vi "pralka.vi"() -> ()   [LabVIEW 2023]
uses:
  cluster.ctl
  states.ctl
panel:
  in  "Lid Open":bool
  in  "Drying Enable":bool
  in  "Start":bool
  in  "Dial":i32(knob)=2 scale=0.0..4.0
  out "Power On":bool
  out "Lid open":bool
  in  "stop":bool
  out "Drying":bool
  out "Centrifugation":bool
  out "Pump water out":bool
  out "Motor controll":bool
  out "Water heating":bool
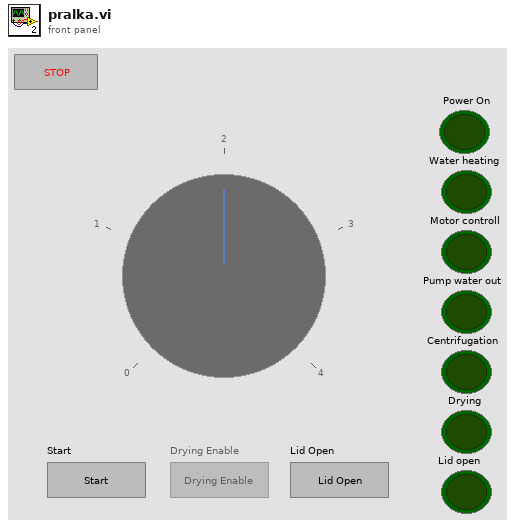
[diagram p1: front panel]
types:
  T1 = typedef "states.ctl" = enum16{"init", "idle", "washing_init", "washing", "wait", "turn_off", "lead_open", "exit"}
  T2 = typedef "cluster.ctl" = cluster{"CurrentTime":timestamp, "CoffeType":enum16{"Cotton", "Silk", "Fast", "Drying"}, "Cluster":cluster{"WaterHeating":i32, "MotorControll":i32, "PumpWaterOut":i32, "Cetrifugation":i32, "Drying":i32}, "TimeToWait":i32, "WashingState":i32, "LidOnTime":dbl}
  T3 = enum8{"Enabled", "Disabled", "Disabled and Grayed Out"}
  T4 = cluster{"WaterHeating":i32, "MotorControll":i32, "PumpWaterOut":i32, "Cetrifugation":i32, "Drying":i32}
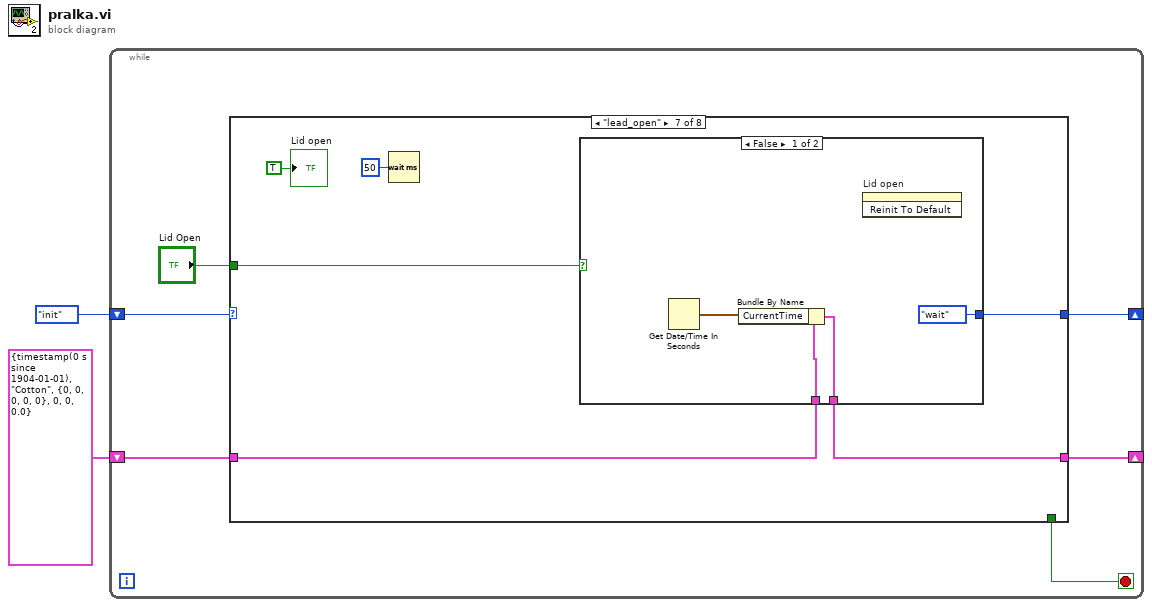
[diagram p0: block diagram]
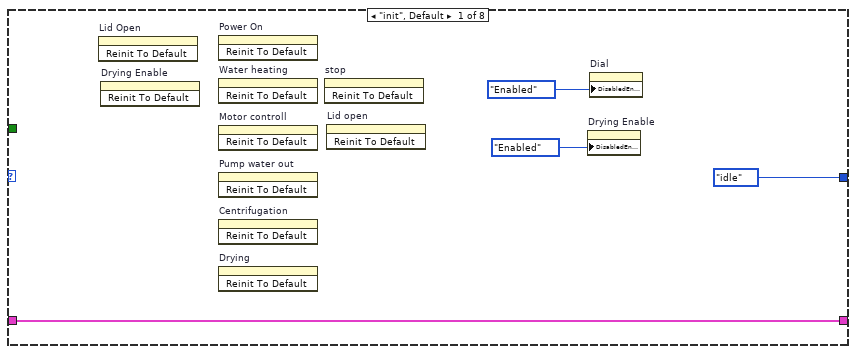
[diagram p2: hidden frame]
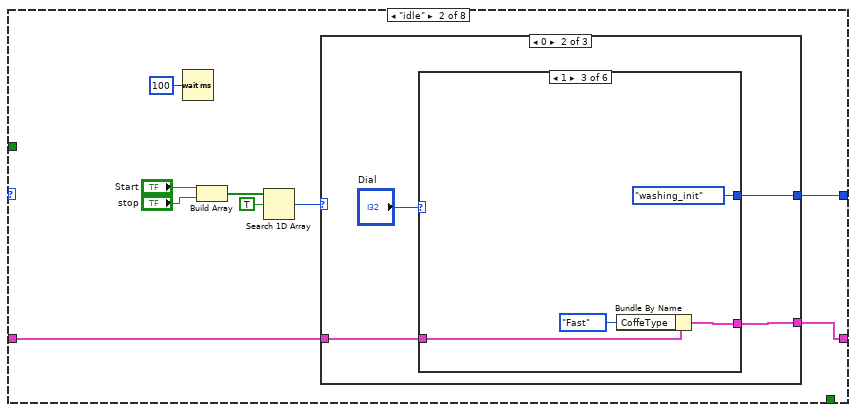
[diagram p3: hidden frame]
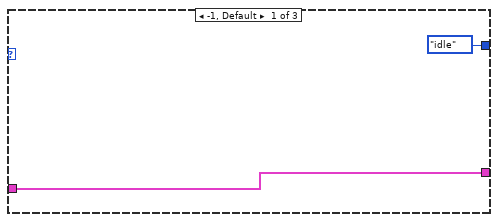
[diagram p4: hidden frame]
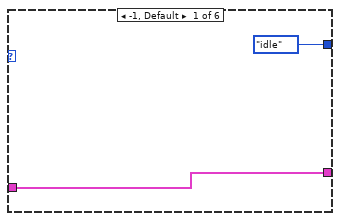
[diagram p5: hidden frame]
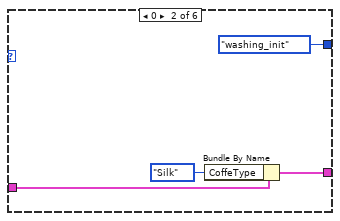
[diagram p6: hidden frame]
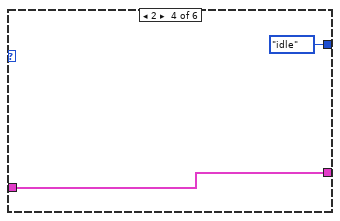
[diagram p7: hidden frame]
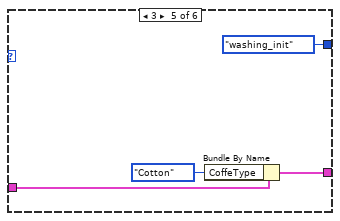
[diagram p8: hidden frame]
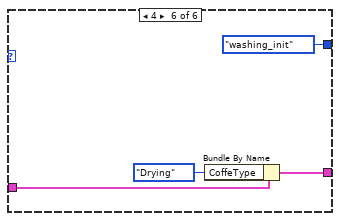
[diagram p9: hidden frame]
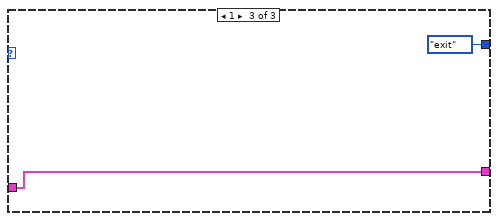
[diagram p10: hidden frame]
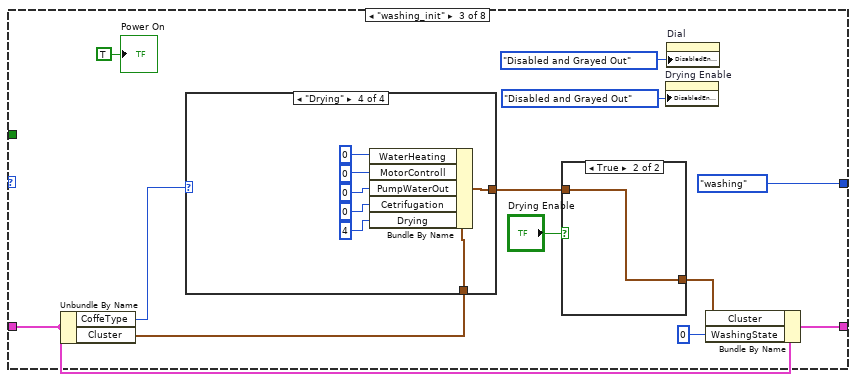
[diagram p11: hidden frame]
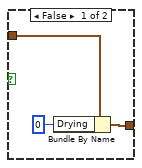
[diagram p12: hidden frame]
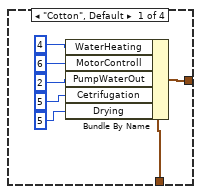
[diagram p13: hidden frame]
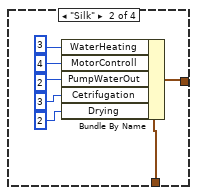
[diagram p14: hidden frame]
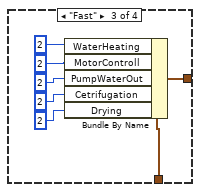
[diagram p15: hidden frame]
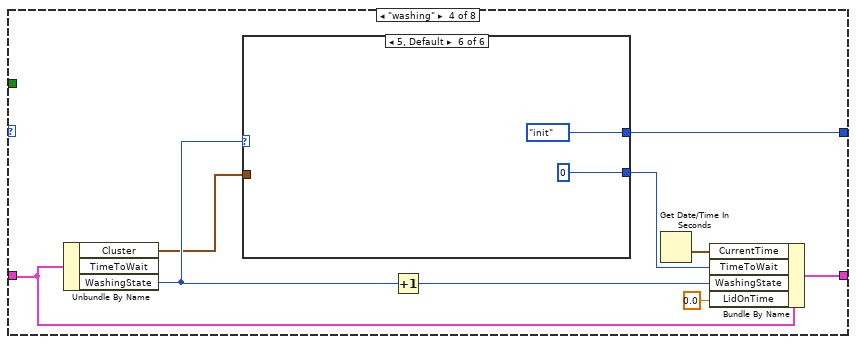
[diagram p16: hidden frame]
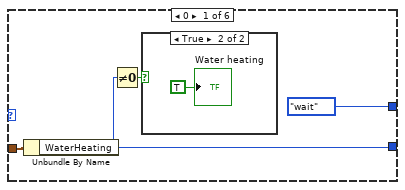
[diagram p17: hidden frame]
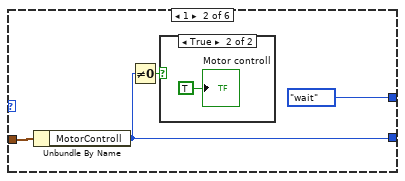
[diagram p19: hidden frame]
diagram:
  n1 = while {
    shift-right: [w7] -> _
    shift-left: states."init" ("Enum") -> [w8]
    shift-right: [w5] -> _
    shift-left: T2 {"CurrentTime"=timestamp(0 s since 1904-01-01), "CoffeType"=enum."Cotton", "Cluster"={"WaterHeating"=0, "MotorControll"=0, "PumpWaterOut"=0, "Cetrifugation"=0, "Drying"=0}, "TimeToWait"=0, "WashingState"=0, "LidOnTime"=0.0} -> [w6]
    stop <- w3 stop-if-true
    n2 = case shown="\"lead_open\"" w8 {
      tunnel: [states."idle" ("Enum") w21 states."washing" ("Enum") w96 w144 states."washing" ("Enum") w174 states."exit" ("Enum")] -> w7
      tunnel: w6 -> [w11 w20 w58 w101 w135 w167 w170 w183]
      tunnel: [w11 w19 w60 w102 w131 w167 w169 w183] -> w5
      tunnel: "Lid Open" -> [_ _ _ _ w136 _ w172 _]
      tunnel: [_ _ _ _ _ _ _ TRUE ("stop")] -> w3
      frame "init", Default {
        n3 = invoke on="Lid Open" class="Bool (strict)" method="Reinit To Default"() -> ()  [unwired: 3 in, 3 out]
        n4 = invoke on="Drying Enable" class="Bool (strict)" method="Reinit To Default"() -> ()  [unwired: 3 in, 3 out]
        n5 = invoke on="Power On" class="Bool (strict)" method="Reinit To Default"() -> ()  [unwired: 3 in, 3 out]
        n6 = invoke on="Water heating" class="Bool (strict)" method="Reinit To Default"() -> ()  [unwired: 3 in, 3 out]
        n7 = invoke on="Motor controll" class="Bool (strict)" method="Reinit To Default"() -> ()  [unwired: 3 in, 3 out]
        n8 = invoke on="Pump water out" class="Bool (strict)" method="Reinit To Default"() -> ()  [unwired: 3 in, 3 out]
        n9 = invoke on="Centrifugation" class="Bool (strict)" method="Reinit To Default"() -> ()  [unwired: 3 in, 3 out]
        n10 = invoke on="Drying" class="Bool (strict)" method="Reinit To Default"() -> ()  [unwired: 3 in, 3 out]
        n11 = invoke on="stop" class="Bool (strict)" method="Reinit To Default"() -> ()  [unwired: 3 in, 3 out]
        n12 = invoke on="Lid open" class="Bool (strict)" method="Reinit To Default"() -> ()  [unwired: 3 in, 3 out]
        n13 = property on="Drying Enable" class="Bool (strict)"("DisabledEnum"=T3."Enabled" ("Disabled")) -> ()  [unwired: 2 in, 2 out]
        n14 = property on="Dial" class="Knob (strict)"("DisabledEnum"=T3."Enabled" ("Disabled")) -> ()  [unwired: 2 in, 2 out]
      }
      frame "idle" {
        n15 = Wait (ms)(milliseconds to wait=u32 100) -> ()  [unwired: 1 out]
        n16 = Build Array("Start", "stop") -> (w15:bool[])
        n17 = Search 1D Array(1D array=w15, element=TRUE) -> (index of element=w13:i32)  [unwired: 1 in]
        n18 = case shown="0" w13 {
          tunnel: [states."idle" ("Enum") w27 states."exit" ("Enum")] -> w21
          tunnel: w20 -> [w22 w26 w49]
          tunnel: [w22 w25 w49] -> w19
          frame -1, Default {
          }
          frame 0 {
            n19 = case shown="1" "Dial" {
              tunnel: [states."idle" ("Enum") states."washing_init" ("Enum") states."washing_init" ("Enum") states."idle" ("Enum") states."washing_init" ("Enum") states."washing_init" ("Enum")] -> w27
              tunnel: w26 -> [w28 w31 w36 w39 w42 w46]
              tunnel: [w28 w32 w37 w39 w43 w47] -> w25
              frame -1, Default {
              }
              frame 0 {
                n20 = Bundle By Name(cluster=w31, "CoffeType"=enum16{"Cotton", "Silk", "Fast", "Drying"}."Silk") -> (w32:T2)
              }
              frame 1 {
                n21 = Bundle By Name(cluster=w36, "CoffeType"=enum16{"Cotton", "Silk", "Fast", "Drying"}."Fast") -> (w37:T2)
              }
              frame 2 {
              }
              frame 3 {
                n22 = Bundle By Name(cluster=w42, "CoffeType"=enum16{"Cotton", "Silk", "Fast", "Drying"}."Cotton") -> (w43:T2)
              }
              frame 4 {
                n23 = Bundle By Name(cluster=w46, "CoffeType"=enum16{"Cotton", "Silk", "Fast", "Drying"}."Drying") -> (w47:T2)
              }
            }
          }
          frame 1 {
          }
        }
      }
      frame "washing_init" {
        n24 = Unbundle By Name(w58) -> ("CoffeType"=w59:enum16{"Cotton", "Silk", "Fast", "Drying"}, "Cluster"=w57:T4)
        n25 = case shown="\"Drying\"" w59 {
          tunnel: [w72 w78 w86 w93] -> w52
          tunnel: w57 -> [w71 w79 w85 w92]
          frame "Cotton", Default {
            n26 = Bundle By Name(cluster=w71, "WaterHeating"=4 ("Espresso"), "MotorControll"=6 ("SteamedMilk"), "PumpWaterOut"=2 ("MilkFoam"), "Cetrifugation"=5 ("ChocolateSyrup"), "Drying"=5 ("WhippedCream")) -> (w72:T4)
          }
          frame "Silk" {
            n27 = Bundle By Name(cluster=w79, "WaterHeating"=3 ("Espresso"), "MotorControll"=4 ("SteamedMilk"), "PumpWaterOut"=2 ("MilkFoam"), "Cetrifugation"=3 ("ChocolateSyrup"), "Drying"=2 ("WhippedCream")) -> (w78:T4)
          }
          frame "Fast" {
            n28 = Bundle By Name(cluster=w85, "WaterHeating"=2 ("Espresso"), "MotorControll"=2 ("SteamedMilk"), "PumpWaterOut"=2 ("MilkFoam"), "Cetrifugation"=2 ("ChocolateSyrup"), "Drying"=2 ("WhippedCream")) -> (w86:T4)
          }
          frame "Drying" {
            n29 = Bundle By Name(cluster=w92, "WaterHeating"=0 ("Espresso"), "MotorControll"=0 ("SteamedMilk"), "PumpWaterOut"=0 ("MilkFoam"), "Cetrifugation"=0 ("ChocolateSyrup"), "Drying"=4 ("WhippedCream")) -> (w93:T4)
          }
        }
        n30 = case shown="True" "Drying Enable" {
          tunnel: [w64 w65] -> w53
          tunnel: w52 -> [w63 w65]
          frame False {
            n31 = Bundle By Name(cluster=w63, "Drying"=0) -> (w64:T4)
          }
          frame True {
          }
        }
        n32 = property on="Drying Enable" class="Bool (strict)"("DisabledEnum"=T3."Disabled and Grayed Out" ("Disabled")) -> ()  [unwired: 2 in, 2 out]
        n33 = property on="Dial" class="Knob (strict)"("DisabledEnum"=T3."Disabled and Grayed Out" ("Disabled")) -> ()  [unwired: 2 in, 2 out]
        n34 = Bundle By Name(cluster=w58, "Cluster"=w53, "WashingState"=0 ("ElementPreparing")) -> (w60:T2)
        "Power On" <- TRUE ("Power On")
      }
      frame "washing" {
        n35 = Unbundle By Name(w101) -> ("Cluster"=w98:T4, "WashingState"=w100:i32)  [unwired: 1 out]
        n36 = case shown="5, Default" w100 {
          tunnel: w98 -> [w106 w111 w116 w121 w126 _]
          tunnel: [w103 w108 w113 w118 w123 0 ("WhippedCream")] -> w97
          tunnel: [states."wait" ("Enum") states."wait" ("Enum") states."wait" ("Enum") states."wait" ("Enum") states."wait" ("Enum") states."init" ("Enum")] -> w96
          frame 0 {
            n37 = Unbundle By Name(w106) -> ("WaterHeating"=w103:i32)
            n38 = Not Equal To 0?(x=w103) -> (x != 0?=w104:bool)
            n39 = case shown="True" w104 {
              frame False {
              }
              frame True {
                "Water heating" <- TRUE ("Espresso")
              }
            }
          }
          frame 1 {
            n40 = Unbundle By Name(w111) -> ("MotorControll"=w108:i32)
            n41 = Not Equal To 0?(x=w108) -> (x != 0?=w109:bool)
            n42 = case shown="True" w109 {
              frame False {
              }
              frame True {
                "Motor controll" <- TRUE ("Steamed Milk")
              }
            }
          }
          frame 2 {
            n43 = Unbundle By Name(w116) -> ("PumpWaterOut"=w113:i32)
            n44 = Not Equal To 0?(x=w113) -> (x != 0?=w114:bool)
            n45 = case shown="True" w114 {
              frame False {
              }
              frame True {
                "Pump water out" <- TRUE ("Milk Foam")
              }
            }
          }
          frame 3 {
            n46 = Unbundle By Name(w121) -> ("Cetrifugation"=w118:i32)
            n47 = Not Equal To 0?(x=w118) -> (x != 0?=w119:bool)
            n48 = case shown="True" w119 {
              frame False {
              }
              frame True {
                "Centrifugation" <- TRUE ("Chocolate Syrup")
              }
            }
          }
          frame 4 {
            n49 = Unbundle By Name(w126) -> ("Drying"=w123:i32)
            n50 = Not Equal To 0?(x=w123) -> (x != 0?=w124:bool)
            n51 = case shown="True" w124 {
              frame False {
              }
              frame True {
                "Drying" <- TRUE ("Whipped Cream")
              }
            }
          }
          frame 5, Default {
          }
        }
        n52 = Increment(x=w100) -> (x+1=w99:i32)
        n53 = Get Date/Time In Seconds() -> (seconds since 1Jan1904=w95:timestamp)
        n54 = Bundle By Name(cluster=w101, "CurrentTime"=w95, "TimeToWait"=w97, "WashingState"=w99, "LidOnTime"=0.0) -> (w102:T2)
      }
      frame "wait" {
        n55 = Unbundle By Name(w135) -> ("CurrentTime"=w142:timestamp, "TimeToWait"=w137:i32, "LidOnTime"=w133:dbl)
        n56 = Get Date/Time In Seconds() -> (seconds since 1Jan1904=w143:timestamp)
        n57 = To Double Precision Float(number=w142) -> (double precision float=w140:dbl)
        n58 = To Double Precision Float(number=w137) -> (double precision float=w139:dbl)
        n59 = To Double Precision Float(number=w143) -> (double precision float=w141:dbl)
        n60 = Subtract(x=w141, y=w140) -> (x-y=w134:dbl)
        n61 = Add(x=w134, y=w133) -> (x+y=w132:dbl)
        n62 = Greater Or Equal?(x=w132, y=w139) -> (x >= y?=w138:bool)
        n63 = local read "stop"() -> (w130:bool)
        n64 = case shown="False" w130 {
          tunnel: [w151 states."exit" ("Enum")] -> w144
          tunnel: w138 -> [w150 _]
          tunnel: w136 -> [w149 _]
          tunnel: w135 -> [w148 w166]
          tunnel: w132 -> [w147 _]
          tunnel: [w146 w166] -> w131
          frame False {
            n65 = case shown="True" w150 {
              tunnel: [w156 states."turn_off" ("Enum")] -> w151
              tunnel: w149 -> [w155 _]
              tunnel: w148 -> [w154 w163]
              tunnel: w147 -> [w153 _]
              tunnel: [w152 w163] -> w146
              frame False {
                n66 = case shown="True" w155 {
                  tunnel: [states."wait" ("Enum") states."lead_open" ("Enum")] -> w156
                  tunnel: w154 -> [w157 w161]
                  tunnel: w153 -> [_ w160]
                  tunnel: [w157 w159] -> w152
                  frame False {
                  }
                  frame True {
                    n67 = Bundle By Name(cluster=w161, "LidOnTime"=w160) -> (w159:T2)
                  }
                }
              }
              frame True {
              }
            }
          }
          frame True {
          }
        }
        n68 = Wait (ms)(milliseconds to wait=u32 100) -> ()  [unwired: 1 out]
      }
      frame "turn_off" {
        n69 = invoke on="Centrifugation" class="Bool (strict)" method="Reinit To Default"() -> ()  [unwired: 3 in, 3 out]
        n70 = invoke on="Water heating" class="Bool (strict)" method="Reinit To Default"() -> ()  [unwired: 3 in, 3 out]
        n71 = invoke on="Pump water out" class="Bool (strict)" method="Reinit To Default"() -> ()  [unwired: 3 in, 3 out]
        n72 = invoke on="Motor controll" class="Bool (strict)" method="Reinit To Default"() -> ()  [unwired: 3 in, 3 out]
        n73 = invoke on="Drying" class="Bool (strict)" method="Reinit To Default"() -> ()  [unwired: 3 in, 3 out]
      }
      frame "lead_open" {
        n74 = Wait (ms)(milliseconds to wait=u32 50) -> ()  [unwired: 1 out]
        n75 = case shown="False" w172 {
          tunnel: [states."wait" ("Enum") states."lead_open" ("Enum")] -> w174
          tunnel: w170 -> [w177 w179]
          tunnel: [w175 w179] -> w169
          frame False {
            n76 = Get Date/Time In Seconds() -> (seconds since 1Jan1904=w176:timestamp)
            n77 = Bundle By Name(cluster=w177, "CurrentTime"=w176) -> (w175:T2)
            n78 = invoke on="Lid open" class="Bool (strict)" method="Reinit To Default"() -> ()  [unwired: 3 in, 3 out]
          }
          frame True {
          }
        }
        "Lid open" <- TRUE ("Lid open")
      }
      frame "exit" {
      }
    }
  }
